vi "getCmd.vi"(8 "error in (no error)":errorcluster, 10 "Name":string, 11 "Subsystem in":refnum<class "Subsystem.lvclass">) -> (0 "error out":errorcluster, 1 "Subsystem Found?":bool, 2 "Command":refnum<class "Command.lvclass">, 3 "Subsystem out":refnum<class "Subsystem.lvclass">)   [LabVIEW 2017, in "Subsystem.lvclass"]
uses:
  <userlib>/836-Library/Robot/Subsystem/Subsystem.lvclass
  <userlib>/836-Library/Robot/Command/Command.lvclass
  <userlib>/836-Library/Robot/Subsystem/Subsystem.lvclass/Subsystem.ctl
  <userlib>/836-Library/Robot/Command/Command.lvclass/Command.ctl
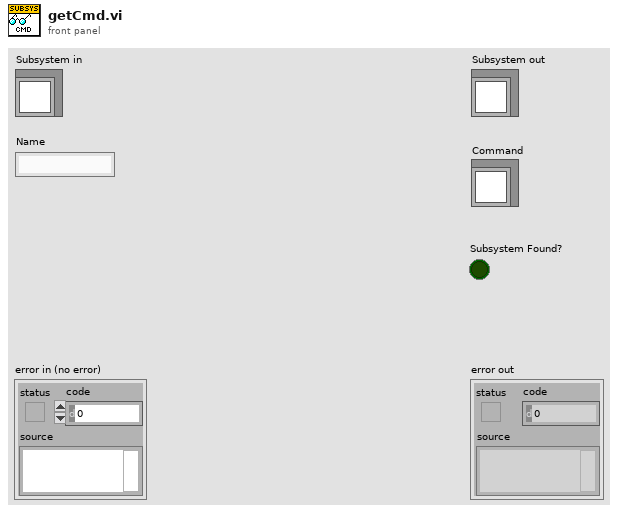
[diagram p1: front panel]
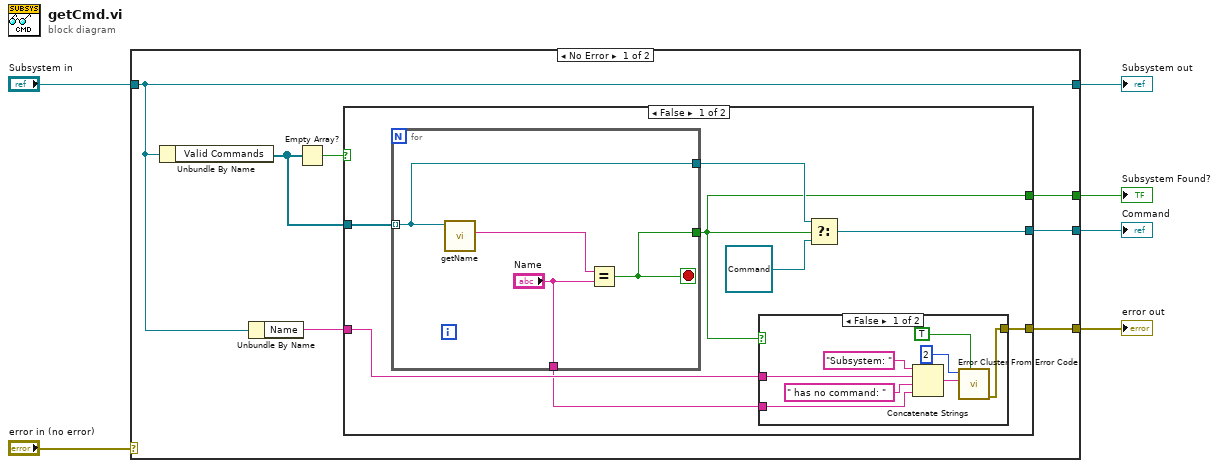
[diagram p0: block diagram]
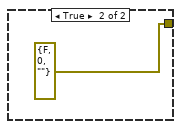
[diagram p2: hidden frame]
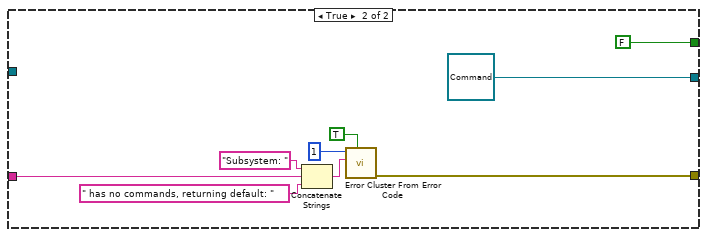
[diagram p3: hidden frame]
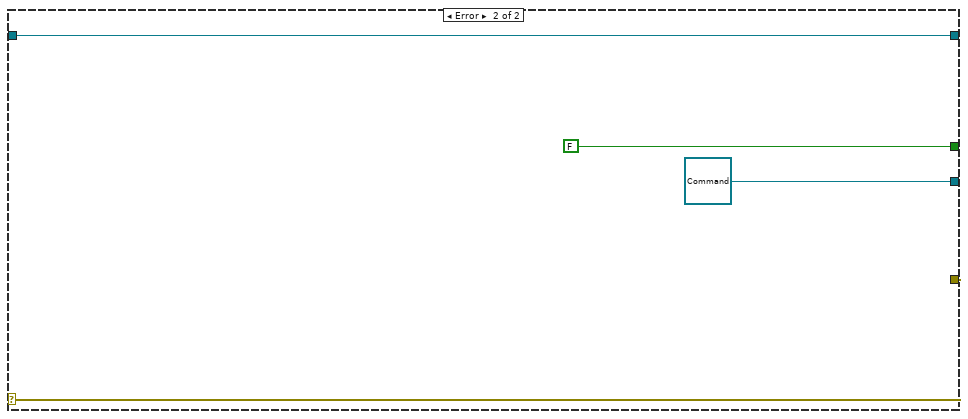
[diagram p4: hidden frame]
diagram:
  n1 = case shown="No Error" "error in (no error)" {
    selector: "error in (no error)" -> [_ w46]
    tunnel: [w9 w46] -> w5
    tunnel: [w11 w47] -> w3
    tunnel: "Subsystem in" -> [w11 w47]
    tunnel: [w12 refnum<class "Command.lvclass"> refnum ("Command.lvclass")] -> w1
    tunnel: [w7 FALSE] -> w2
    frame No Error {
      n2 = Unbundle By Name(w11) -> ("Valid Commands"=w10:refnum<class "Command.lvclass">[])
      n3 = Unbundle By Name(w11) -> ("Name"=w8:string)
      n4 = Empty Array?(array=w10) -> (empty?=w13:bool)
      n5 = case shown="False" w13 {
        tunnel: [w19 refnum<class "Command.lvclass"> refnum ("Command.lvclass")] -> w12
        tunnel: w10 -> [w21 _]
        tunnel: [w18 w38] -> w9
        tunnel: w8 -> [w16 w37]
        tunnel: [w17 FALSE] -> w7
        frame False {
          n6 = for {
            tunnel: w21 -> [w32] mode=indexing
            tunnel: [w34] -> w17
            tunnel: [w32] -> w20
            tunnel: ["Name"] -> w15
            stop <- w34 stop-if-true
            n7 = call <userlib>:"getName.vi"("Command in"=w32) -> ("Name"=w31:string)  [unwired: 8 in, 2 out]
            n8 = Equal?(x=w31, y="Name") -> (x = y?=w34:bool)
          }
          n9 = case shown="False" w17 {
            tunnel: [w29 errorcluster {"status"=FALSE, "code"=0, "source"=""} ("error out")] -> w18
            tunnel: w16 -> [w25 _]
            tunnel: w15 -> [w23 _]
            frame False {
              n10 = Concatenate Strings("Subsystem: ", w25, " has no command: " ("string"), w23) -> (w22:string)
              n11 = call <vilib>:"Error Cluster From Error Code.vi"("show call chain? (False)"=TRUE, "error message (\"\")"=w22, "error code (0)"=2) -> ("error out"=w29:errorcluster)  [unwired: 6 in]
            }
            frame True {
            }
          }
          n12 = Select(t=w20, s=w17, f=refnum<class "Command.lvclass"> refnum ("Command.lvclass")) -> (s? t:f=w19:refnum<class "Command.lvclass">)
        }
        frame True {
          n13 = Concatenate Strings("Subsystem: ", w37, " has no commands, returning default: ") -> (w41:string)
          n14 = call <vilib>:"Error Cluster From Error Code.vi"("show call chain? (False)"=TRUE, "error message (\"\")"=w41, "error code (0)"=1) -> ("error out"=w38:errorcluster)  [unwired: 6 in]
        }
      }
    }
    frame Error {
    }
  }
  "error out" <- w5
  "Subsystem out" <- w3
  "Subsystem Found?" <- w2
  "Command" <- w1
